vi "Shutdown.vi"(8 "error in (no error)":errorcluster, 11 "Camera in":refnum<class "Camera.lvclass">) -> (0 "error out":errorcluster, 3 "Camera out":refnum<class "Camera.lvclass">)   [LabVIEW 2020, in "Camera.lvlib" / "Camera.lvclass"]
uses:
  Camera.lvclass
  Camera.lvclass/Camera.ctl
  Device/Device/Device.lvclass
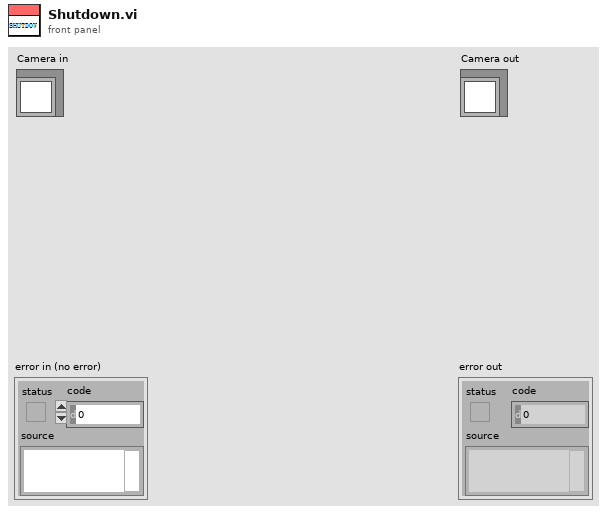
[diagram p1: front panel]
types:
  T1 = typedef "IMAQ Image.ctl" = refnum<image>
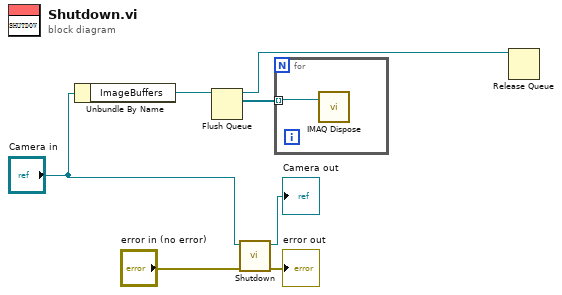
[diagram p0: block diagram]
diagram:
  n1 = Unbundle By Name("Camera in") -> ("ImageBuffers"=w3:refnum<queue>)
  n2 = Flush Queue(queue=w3) -> (queue out=w1:refnum<queue>, remaining elements=w2:T1[])  [unwired: 1 in, 1 out]
  n3 = call-parent "Shutdown.vi"("error in (no error)"="error in (no error)", "Device in"="Camera in") -> ("error out"=→"error out":errorcluster, "Device out"=→"Camera out":refnum<class "Camera.lvclass">)  [unwired: 8 in]
  n4 = for {
    tunnel: w2 -> [w8] mode=indexing
    n5 = call "IMAQ Dispose"("Image"=w8) -> ()  [unwired: 5 in, 1 out]
  }
  n6 = Release Queue(queue=w1) -> ()  [unwired: 2 in, 3 out]
